vi "get last camera data.vi"(7 "Now":timestamp, 8 "life time":dbl, 9 "camera_id":u32, 11 "Detection Frame In":T2) -> (3 "output array":T1(array[cluster]))   [LabVIEW 2016]
uses:
  GitHub/SSLView/SSL Detection Frame.ctl
  GitHub/SSLView/SSL Detection Robot.ctl
  GitHub/SSLView/SSL Detection Ball.ctl
panel:
  # "recebe os dados de uma câmera, armazena apenas o mais recente"
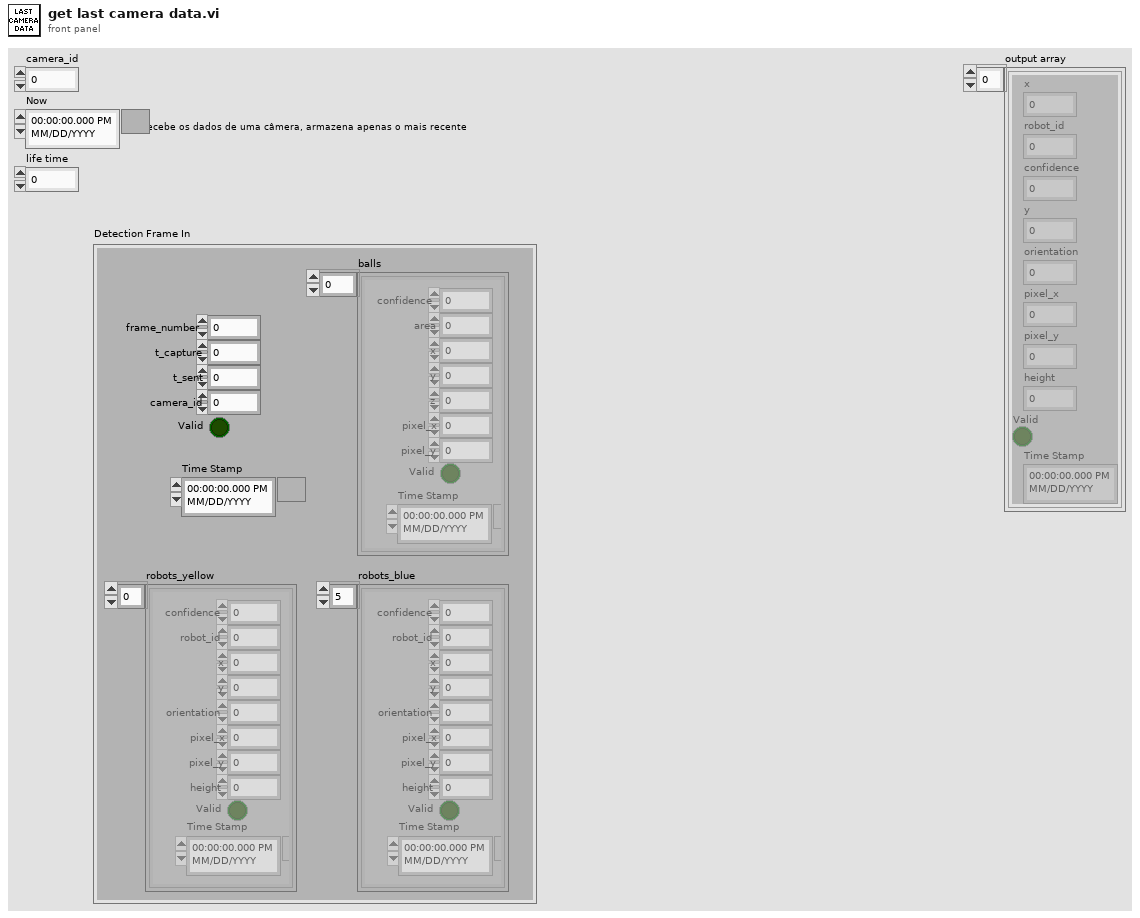
[diagram p1: front panel]
types:
  T1 = cluster{"x":dbl, "robot_id":u32, "confidence":sgl, "y":sgl, "orientation":sgl, "pixel_x":sgl, "pixel_y":sgl, "height":sgl, "Valid":bool, "Time Stamp":timestamp}[]
  T2 = typedef "SSL Detection Frame.ctl" = cluster{"frame_number":u32, "t_capture":dbl, "t_sent":dbl, "camera_id":u32, "robots_yellow":T3[], "robots_blue":T3[], "balls":T4[], "Valid":bool, "Time Stamp":timestamp}
  T3 = typedef "SSL Detection Robot.ctl" = cluster{"x":dbl, "robot_id":u32, "confidence":sgl, "y":sgl, "orientation":sgl, "pixel_x":sgl, "pixel_y":sgl, "height":sgl, "Valid":bool, "Time Stamp":timestamp}
  T4 = typedef "SSL Detection Ball.ctl" = cluster{"x":sgl, "area":u32, "confidence":sgl, "y":sgl, "z":sgl, "pixel_x":sgl, "pixel_y":sgl, "Valid":bool, "Time Stamp":timestamp}
  T5 = cluster{"x":dbl, "robot_id":u32, "confidence":sgl, "y":sgl, "orientation":sgl, "pixel_x":sgl, "pixel_y":sgl, "height":sgl, "Valid":bool, "Time Stamp":timestamp}
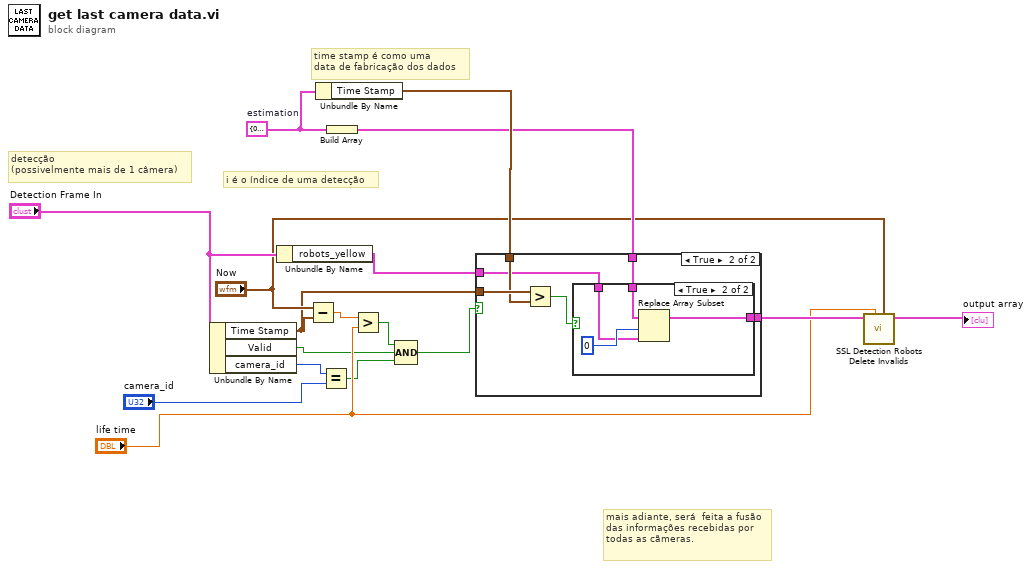
[diagram p0: block diagram]
diagram:
  w13 = T5 {"x"=0.0, "robot_id"=0, "confidence"=0.0, "y"=0.0, "orientation"=0.0, "pixel_x"=0.0, "pixel_y"=0.0, "height"=0.0, "Valid"=FALSE, "Time Stamp"=timestamp(0 s since 1904-01-01)}  # estimation
  # "i é o índice de uma detecção"
  # "time stamp é como uma\ndata de fabricação dos dados"
  # "mais adiante, será  feita a fusão das informações recebidas por todas as cãmeras."
  # "detecção\n(possivelmente mais de 1 câmera)"
  n1 = Unbundle By Name("Detection Frame In") -> ("Time Stamp"=w3:timestamp, "Valid"=w6:bool, "camera_id"=w8:u32)
  n2 = Unbundle By Name("Detection Frame In") -> ("robots_yellow"=w1:T3[])
  n3 = Subtract(x="Now", y=w3) -> (x-y=w5:dbl)
  n4 = Unbundle By Name(w13) -> ("Time Stamp"=w15:timestamp)
  n5 = Equal?(x=w8, y="camera_id") -> (x = y?=w7:bool)
  n6 = Build Array(w13) -> (w14:T1)
  n7 = Greater?(x=w5, y="life time") -> (0:w4:bool)
  n8 = Compound Arithmetic op=AND(w4, w6, w7) -> (w2:bool)
  n9 = case shown="True" w2 {
    tunnel: w15 -> [_ w22]
    tunnel: w3 -> [_ w24]
    tunnel: w14 -> [w18 w21]
    tunnel: w1 -> [_ w20]
    tunnel: [w18 w19] -> w11
    frame False {
    }
    frame True {
      n10 = Greater?(x=w24, y=w22) -> (0:w23:bool)
      n11 = case shown="True" w23 {
        tunnel: w21 -> [w25 w29]
        tunnel: w20 -> [_ w27]
        tunnel: [w25 w26] -> w19
        frame False {
        }
        frame True {
          n12 = Replace Array Subset(array=w29, new element=w27, index=0) -> (w26:T1)
        }
      }
    }
  }
  n13 = call "SSL Detection Robots Delete Invalids.vi"("Now"="Now", "Life Time"="life time", "Robots In"=w11) -> ("Robots Out"=→"output array":T3[])  [unwired: 8 in]
